vi "Error 6004.vi"(8 "error in (no error)":errorcluster, 10 "datatype":string) -> (0 "error out":errorcluster)   [LabVIEW 2018, in "Scalar IO Operations.lvlib"]
uses:
  Scalar IO Operations.lvlib
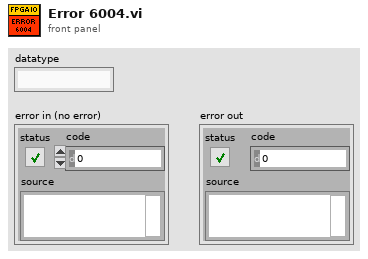
[diagram p1: front panel]
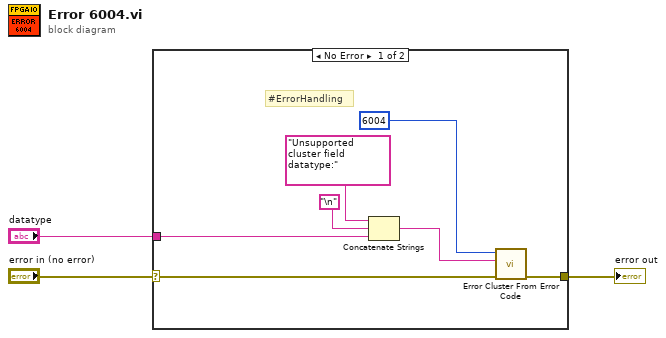
[diagram p0: block diagram]
diagram:
  n1 = case shown="No Error" "error in (no error)" {
    selector: "error in (no error)" -> [w5 w11]
    tunnel: "datatype" -> [w8 _]
    tunnel: [w6 w11] -> w2
    frame No Error {
      # "#ErrorHandling"
      n2 = Concatenate Strings("Unsupported cluster field datatype:" ("error message (\"\")"), "\n", w8) -> (w9:string)
      n3 = call <vilib>:"Error Cluster From Error Code.vi"("error in (no error)"=w5, "error message (\"\")"=w9, "error code (0)"=6004) -> ("error out"=w6:errorcluster)  [unwired: 6 in]
    }
    frame Error {
    }
  }
  "error out" <- w2
